vi "OpenShortDeembed_Read_and_Write_SnP_Files.vi"() -> ()   [LabVIEW 2021]
uses:
  Program Files (x86)/National Instruments/LabVIEW 2020/vi.lib/addons/HF Network Analysis/Support VIs/Read SnP File (SnP).vi
  Program Files (x86)/National Instruments/LabVIEW 2020/vi.lib/addons/HF Network Analysis/NI_HFNetworkAnalysis.lvlib
panel:
  out "S-parameters":cdb[][](array[numeric]) format="%#.6g"
  out "Error Out":errorcluster
  out "Z0 (Ohm)":cdb
  out "Frequencies (Hz)":dbl[](array[numeric])
  in  "Error In":errorcluster
  in  "SnP File Path":path
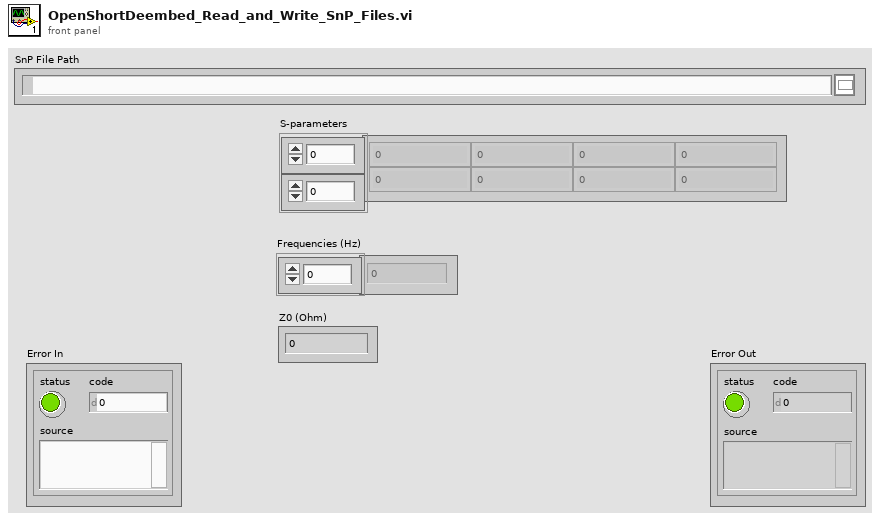
[diagram p1: front panel]
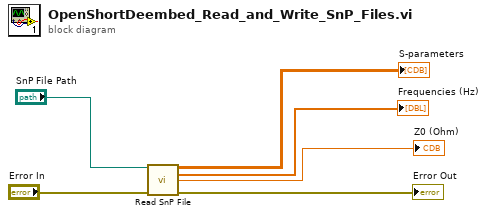
[diagram p0: block diagram]
diagram:
  n1 = call-poly "Read SnP File.vi"("SnP File Path"="SnP File Path", "Error In"="Error In") -> ("S-parameters"=→"S-parameters":cdb[][], "Frequencies (Hz)"=→"Frequencies (Hz)":dbl[], "Z0 (Ohm)"=→"Z0 (Ohm)":cdb, "Error Out"=→"Error Out":errorcluster)  [unwired: 10 in]
